vi "Get log file name.vi"() -> (3 "log file name":string)   [LabVIEW 2018]
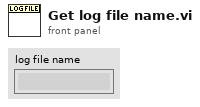
[diagram p1: front panel]
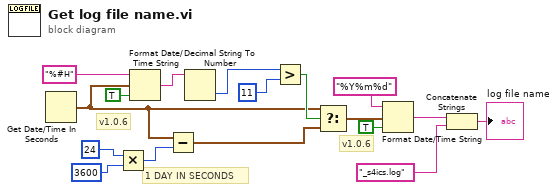
[diagram p0: block diagram]
diagram:
  # "v1.0.6"
  # "v1.0.6"
  # "1 DAY IN SECONDS"
  n1 = Get Date/Time In Seconds() -> (seconds since 1Jan1904=w7:timestamp)
  n2 = Multiply(x=24, y=3600) -> (x*y=w9:i32)
  n3 = Format Date/Time String(time format string (%c)="%#H", seconds (now)=w7, UTC format=TRUE) -> (date/time string=w14:string)
  n4 = Subtract(x=w7, y=w9) -> (x-y=w6:timestamp)
  n5 = Decimal String To Number(string=w14) -> (number=w13:i32)  [unwired: 2 in, 1 out]
  n6 = Greater?(x=w13, y=11) -> (0:w8:bool)
  n7 = Select(t=w7, s=w8, f=w6) -> (s? t:f=w5:timestamp)
  n8 = Format Date/Time String(time format string (%c)="%Y%m%d", seconds (now)=w5, UTC format=TRUE) -> (date/time string=w4:string)
  n9 = Concatenate Strings(w4, "_s4ics.log" ("string")) -> (→"log file name":string)
